vi "Leybold TURBOVAC Access Parameters.vi"() -> ()   [LabVIEW 2019]
doc: "Example VI to demonstrate the use of the Oerlikon Leybold TMP driver."
uses:
  <instrlib>/Leybold TURBOVAC/Public/Ctl/Converter Type Control.ctl
  <instrlib>/Leybold TURBOVAC/Leybold TURBOVAC.lvlib
panel:
  in  "Converter Type\n(180: Turbovac 350/450 i)":T1=187 items=["Turbovac 350/450 i"=180, "Turbovac 350/450 i with optional interface"=181, "Turbovac 350/450 iX"=182, "Turbovac 90/250 i"=190, "Turbovac 90/250 with optional interface"=191, "Turbovac 90/250 iX"=192, "TURBOVAC 850/950 i"=195, "TURBOVAC 850/950 i with optional interface"=196, "TURBOVAC 850/950 iX"=197, "TURBOVAC 1300 i"=185, "TURBOVAC 1300 i with optional interface"=186, "TURBOVAC 1300 iX"=187]
  in  "Type of parameter access (2)":u8(ring) items=["Do nothing"=0, "Parameter value"=1, "Write 16 bit value"=2, "Write 32 bit value"=3, "Field value requested"=6, "Write 16 bit field value"=7, "Write 32 bit field value"=8, "Request No. of field elements"=9]
  out "PWE out":i32
  in  "PWE (0)":i32
  in  "Index (0)":u16 step=1
  in  "PKE-PM No. (1)":u16=1 min=1 step=1
  in  "Converter address (0)":u8
  in  "VISA resource name":refnum<visa-resource-name>="COM43"
  # "© 2020 Leybold.  ALL RIGHTS RESERVED."
  # "Refer to converter manual for the\nvariable size of the parameter to write. Default\nis a 16 bit value.\nSelect \"Do nothing\" to read a parameter only."
  # "Parameter number according to manual."
  # "Some paramters access array of values.\nUse index to access a specific value."
  # "Parameter value to write."
  # "Value as received from the converter according to the settings in PKE-PM No. and Index:"
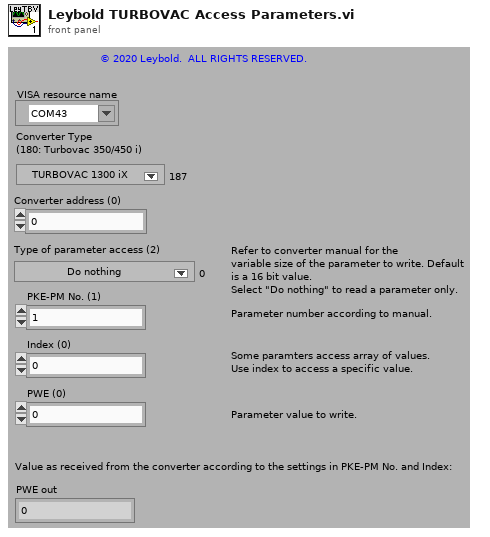
[diagram p1: front panel]
types:
  T1 = typedef "Leybold TURBOVAC.lvlib/Converter Type Control.ctl" = u16
  T2 = typedef "Leybold TURBOVAC.lvlib/Device Parameters Indicator.ctl" = cluster{"Length of data block":u8, "Converter address":u8, "Converter type":T3, "PZD1":u16, "PZD2":u16}
  T3 = typedef "Leybold TURBOVAC.lvlib/Converter Type Indicator.ctl" = u16
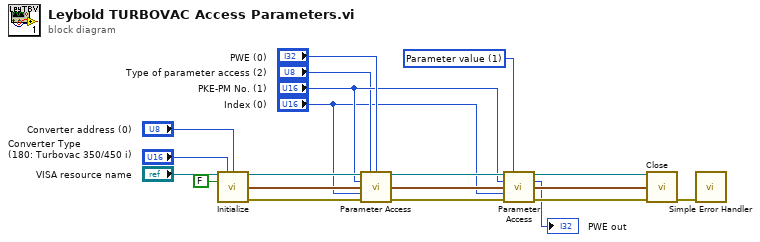
[diagram p0: block diagram]
diagram:
  w7 = u8 1 items=["Do nothing"=0, "Parameter value"=1, "Write 16 bit value"=2, "Write 32 bit value"=3, "Field value requested"=6, "Write 16 bit field value"=7, "Write 32 bit field value"=8, "Request No. of field elements"=9] ("Type of parameter access (1: Parameter value)")
  n1 = call <instrlib>:"Initialize.vi"("VISA resource name"="VISA resource name", "Converter Type\n(180: Turbovac 350/450 i)"="Converter Type\n(180: Turbovac 350/450 i)", "Converter address (0)"="Converter address (0)", "ID Query? (T: Yes)"=FALSE) -> ("VISA resource name out"=w8:refnum<visa-resource-name>, "Device parameters out"=w12:T2, "error out"=w11:errorcluster)  [unwired: 9 in]
  n2 = call <instrlib>:"Parameter Access.vi"("VISA resource name"=w8, "Type of parameter access (1: Parameter value)"="Type of parameter access (2)", "PWE (0)"="PWE (0)", "PKE-PM No. (1)"="PKE-PM No. (1)", "Device parameters"=w12, "Index (0)"="Index (0)", "error in (no error)"=w11) -> ("VISA resource name out"=w9:refnum<visa-resource-name>, "Device parameters out"=w13:T2, "error out"=w10:errorcluster)  [unwired: 5 in, 1 out]
  n3 = call <instrlib>:"Parameter Access.vi"("VISA resource name"=w9, "Type of parameter access (1: Parameter value)"=w7, "PKE-PM No. (1)"="PKE-PM No. (1)", "Device parameters"=w13, "Index (0)"="Index (0)", "error in (no error)"=w10) -> ("VISA resource name out"=w15:refnum<visa-resource-name>, "PWE out"=→"PWE out":i32, "Device parameters out"=w14:T2, "error out"=w16:errorcluster)  [unwired: 6 in]
  n4 = call <instrlib>:"Close.vi"("VISA resource name"=w15, "Device Parameters"=w14, "error in (no error)"=w16) -> ("error out"=w19:errorcluster)  [unwired: 12 in]
  n5 = call <vilib>:"Simple Error Handler.vi"("error in (no error)"=w19) -> ()  [unwired: 4 in, 5 out]
